vi "Reject negative rel times.vi"(10 "Timestamps (ms)":dbl[](array[numeric])) -> (3 "Keep":bool[](array[boolean]))   [LabVIEW 2020]
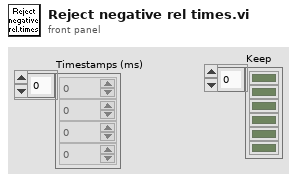
[diagram p1: front panel]
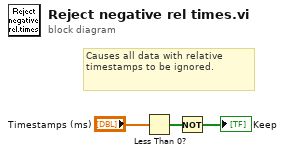
[diagram p0: block diagram]
diagram:
  # "Causes all data with relative timestamps to be ignored."
  n1 = Less Than 0?(x="Timestamps (ms)") -> (x < 0?=w2:bool[])
  n2 = Not(x=w2) -> (.not. x?=→"Keep":bool[])
